vi "mecanum-drive-pose-est-test.vi"(8 "error in (no error)":errorcluster) -> (0 "error out":errorcluster, 3 "Test Passed":bool)   [LabVIEW 2019]
uses:
  <vilib>/Rock Robotics/WPI/ThirdParty/JAS_Junk/TrajLib/MatBuilder_Create.vi
  <vilib>/Rock Robotics/WPI/ThirdParty/JAS_Junk/TrajLib/MatrixHelper_CoerceSize.vi
  <vilib>/Rock Robotics/WPI/ThirdParty/JAS_Junk/TrajLib/Util_CalcDist.vi
  <vilib>/Analysis/1siggen.llb/Gaussian White Noise.vi
  <vilib>/Rock Robotics/WPI/ThirdParty/JAS_Junk/TrajLib/Trajectory_Library.lvlib
panel:
  out "Upd Err":bool
  out "BenchProcessing Timer Per Pass":dbl
  out "BenchTotalTime":dbl
  out "BenchTotalPasses":dbl
  out "MaxErrPassed":bool
  out "TotalPassed":bool
  out "EerrSumNormalized":dbl
  out "Error Sum":dbl
  out "Max Error":dbl
  out "Using Vision":bool
  in  "UseVIsion":bool=TRUE
  out "VIsionUpdates":i32
  out "TotalTImeSecs":dbl
  out "Position Graph":cluster{dbl[], dbl[]}[](graph)
  out "PoesEstCreateErr":errorcluster
  # "< 0.125"
  # "< 0.05"
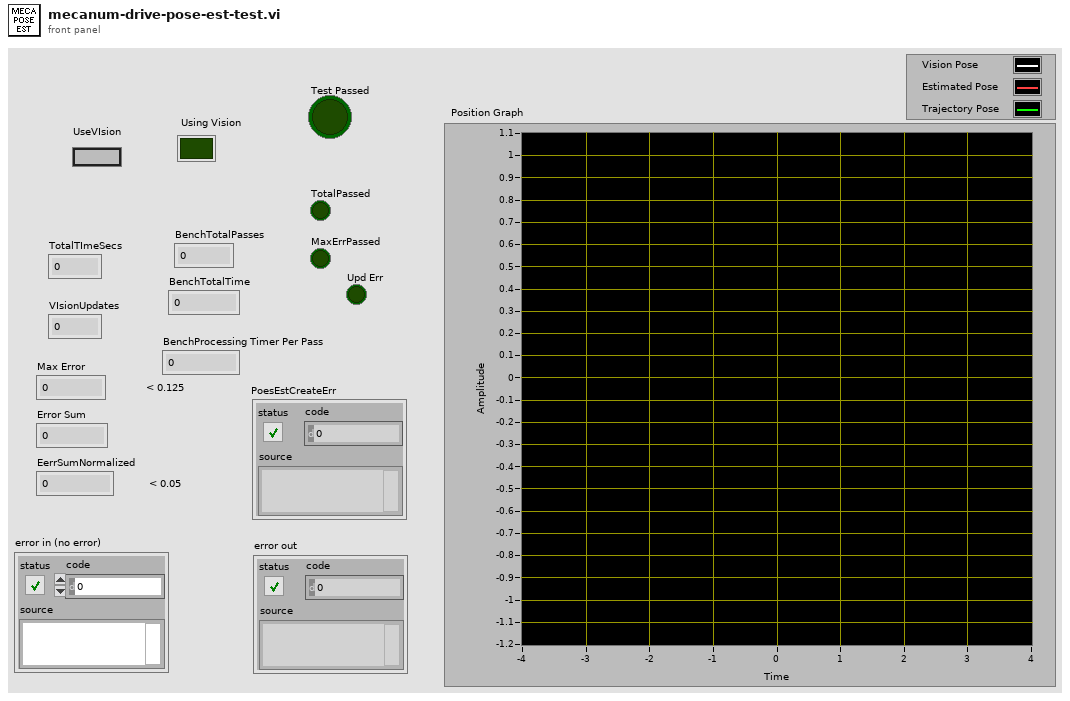
[diagram p1: front panel]
types:
  T1 = typedef "Trajectory_Library.lvlib/TRANSLATION2D.ctl" = cluster{"X":dbl, "Y":dbl}
  T2 = typedef "Trajectory_Library.lvlib/MECA_WHEEL_POSITIONS.ctl" = cluster{"FrontLeft":dbl, "FrontRight":dbl, "RearLeft":dbl, "RearRight":dbl, "P":bool}
  T3 = typedef "Trajectory_Library.lvlib/ROTATION2D.ctl" = cluster{"VALUE":dbl, "COS":dbl, "SIN":dbl}
  T4 = typedef "Trajectory_Library.lvlib/POSE2D.ctl" = cluster{"TRANSLATION":T1, "ROTATION":T3}
  T5 = typedef "NI_Matrix.lvlib/RealMatrix.ctl" = dbl[][]
  T6 = typedef "Trajectory_Library.lvlib/MECA_DRIVE_KINEMATICS.ctl" = cluster{"FrontLeft":T1, "FrontRight":T1, "RearLeft":T1, "RearRight":T1, "InverseKinematics":T5, "ForwardKinematics":T5, "PrevCoR":T1}
  T7 = typedef "Trajectory_Library.lvlib/TRAJ_CONFIG.ctl" = cluster{"MaxVelocity":dbl, "Max Acceleration":dbl, "StartVelocity":dbl, "End Velocity":dbl, "Reversed":bool, "Constraints":variant[]}
  T8 = typedef "Trajectory_Library.lvlib/MECA_DRIVE_POSE_EST.ctl" = cluster{"M_VisionContR":T5, "m_nominal_dT":dbl, "m_PrevTime_Sec":dbl, "m_GyroOffset":T3, "m_PrevAngle":T3, "m_Observer":T9, "m_kinematics":T6, "Pose_Buffer":T12}
  T9 = typedef "Trajectory_Library.lvlib/UNSCENTED_KALMAN_FILTER.ctl" = cluster{"m_P":T5, "m_xHat":T5, "States":i32, "Outputs":i32, "m_ContR":T5, "m_ContQ":T5, "m_SigmasF":T5, "m_dT_Sec":dbl, "MERWE_SCALED_SIGMA_PTS":T10, "meanFuncX":T11, "meanFuncY":T11, "residualFuncX":T11, "residualFuncY":T11, "addFuncX":T11, "addFuncXExtra":variant, "residualFuncYExtra":variant, "residualFuncXExtra":variant, "MeanFuncYExtra":variant, "MeanFuncXExtra":variant, "Inputs":i32}
  T10 = typedef "Trajectory_Library.lvlib/MERWE_SCALED_SIGMA_PTS.ctl" = cluster{"m_Wm":T5, "States":i32, "Alpha":dbl, "m_Wc":T5, "Kappa":i32}
  T11 = typedef "Trajectory_Library.lvlib/CALLBACK_FUNC_TYPE.ctl" = refnum<vi>
  T12 = typedef "Trajectory_Library.lvlib/TIME_INTERPOLATABLE_POSE2D.ctl" = cluster{"TimeStamps":dbl[], "Pose":T4[], "Min_TimeStamp":dbl, "Max_TimeStamp":dbl, "ItemCount":i32, "MaxBufferTime":dbl}
  T13 = typedef "Trajectory_Library.lvlib/TRAJECTORY.ctl" = cluster{"TotalTImeSecs":dbl, "States":T14[]}
  T14 = typedef "Trajectory_Library.lvlib/TRAJ_STATE.ctl" = cluster{"TimeSeconds":dbl, "Velocity":dbl, "Acceleration":dbl, "POSE":T4, "Curvature":dbl}
  T15 = typedef "Trajectory_Library.lvlib/CHASSIS_SPEEDS.ctl" = cluster{"vX":dbl, "vY":dbl, "vOmega":dbl}
  T16 = typedef "Trajectory_Library.lvlib/MECA_WHEEL_SPEEDS.ctl" = cluster{"FrontLeftSpeed":dbl, "FrontRightSpeed":dbl, "RearLeftSpeed":dbl, "RearRightSpeed":dbl}
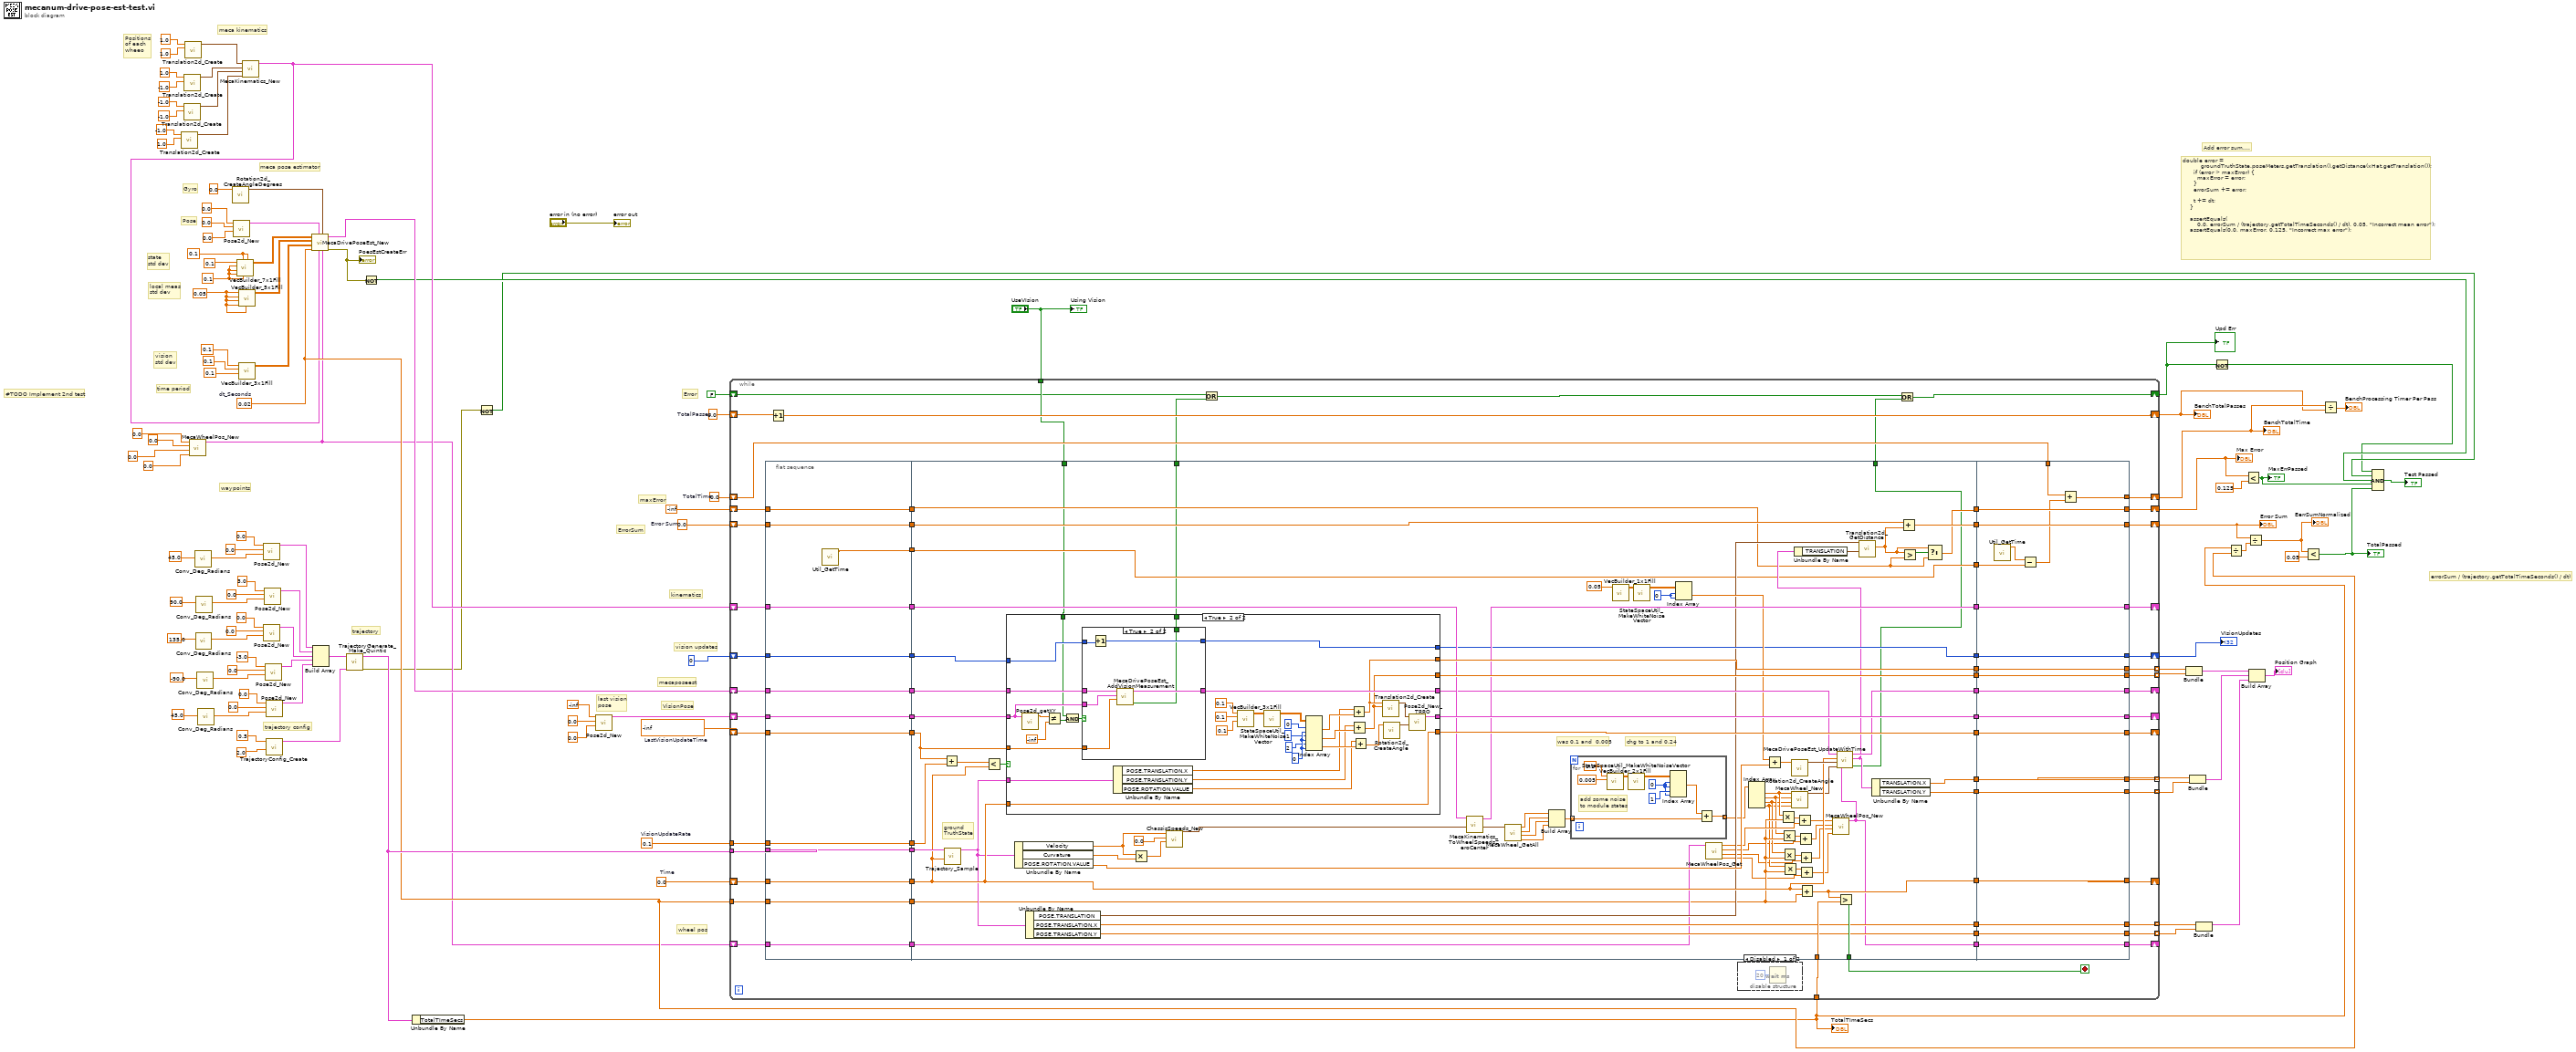
[diagram p0: block diagram]
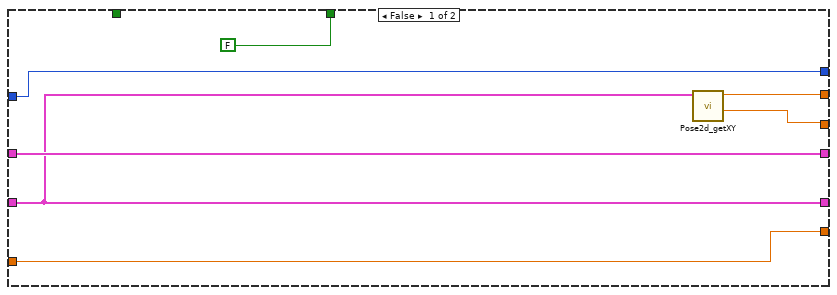
[diagram p3: hidden frame]
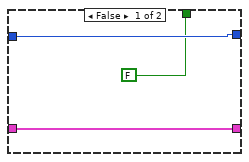
[diagram p4: hidden frame]
diagram:
  w24 = 0.0  # TotalPasses
  w25 = 0.0  # TotalTime
  w37 = 0.0  # Error Sum
  w55 = 0.1  # VisionUpdateRate
  w56 = -inf  # LastVisionUpdateTime
  w58 = 0.0  # Time
  w35 = 0.02  # dt_Seconds
  w8 = 0.05 ("element")
  w9 = 0.1 ("element")
  w11 = 0.1 ("element")
  # "#TODO Implement 2nd test"
  # "errorSum / (trajectory.getTotalTimeSeconds() / dt)"
  # "Error"
  # "Add error sum...."
  # "double error =\n          groundTruthState.poseMeters.getTranslation().getDistance(xHat.getTranslation());\n      if (error > maxError) {\n        maxError = error;\n      }\n      errorSum += error;\n\n      t += dt;\n    }\n\n    assertEquals(\n        0.0, errorSum / (trajectory.getTotalTimeSeconds() / dt), 0.05, \"Incorrect mean error\");\n    assertEquals(0.0, maxError, 0.125, \"Incorrect max error\");"
  # "wheel pos"
  # "ErrorSum"
  # "maxError"
  # "vision updates"
  # "kinematics"
  # "mecaposeest"
  # "VisionPose"
  # "last vision\npose"
  # "time period"
  # "vision \nstd dev"
  # "local meas\nstd dev"
  # "state\nstd dev"
  # "Pose"
  # "Gyro"
  # "Positions\nof each\nwheeo"
  # "meca pose estimator"
  # "meca kinematics"
  # "trajectory config"
  # "trajectory"
  # "waypoints"
  n1 = call <vilib>:"Translation2d_Create.vi"("Y"=1.0, "X"=-1.0) -> ("TRANSLATION"=w71:T1)  [unwired: 9 in]
  n2 = call <vilib>:"Translation2d_Create.vi"("Y"=-1.0, "X"=-1.0) -> ("TRANSLATION"=w72:T1)  [unwired: 9 in]
  n3 = call <vilib>:"Translation2d_Create.vi"("Y"=-1.0, "X"=1.0) -> ("TRANSLATION"=w73:T1)  [unwired: 9 in]
  n4 = call <vilib>:"Translation2d_Create.vi"("Y"=1.0, "X"=1.0) -> ("TRANSLATION"=w74:T1)  [unwired: 9 in]
  n5 = call <vilib>:"MecaWheelPos_New.vi"("RearRightPosition"=0.0, "RearLeftPosition"=0.0, "FrontRightPosition"=0.0, "FrontLeftPosition"=0.0) -> ("MECA_WHEEL_POSITIONS"=w12:T2)  [unwired: 7 in]
  n6 = call <vilib>:"Conv_Deg_Radians.vi"("Degress"=45.0 ("Heading")) -> ("Radians"=w88:dbl)  [unwired: 10 in]
  n7 = call <vilib>:"Conv_Deg_Radians.vi"("Degress"=135.0 ("Heading")) -> ("Radians"=w96:dbl)  [unwired: 10 in]
  n8 = call <vilib>:"Conv_Deg_Radians.vi"("Degress"=90.0 ("Heading")) -> ("Radians"=w92:dbl)  [unwired: 10 in]
  n9 = call <vilib>:"Conv_Deg_Radians.vi"("Degress"=-90.0 ("Heading")) -> ("Radians"=w100:dbl)  [unwired: 10 in]
  n10 = call <vilib>:"Conv_Deg_Radians.vi"("Degress"=45.0 ("Heading")) -> ("Radians"=w104:dbl)  [unwired: 10 in]
  n11 = call <vilib>:"Rotation2d_CreateAngleDegrees.vi"("Angle_Degrees"=0.0) -> ("ROTATION"=w70:T3)  [unwired: 10 in]
  n12 = call <vilib>:"Pose2d_New.vi"("Heading"=0.0, "Y"=0.0, "X"=0.0) -> ("out POSe"=w68:T4)  [unwired: 8 in]
  n13 = call <vilib>:"VecBuilder_7x1Fill.vi"("R0"=w11, "R6"=w9, "R1"=w11, "R5"=w9, "R4"=w9, "R3"=w9, "R2"=0.1 ("element")) -> ("output matrix"=w64:T5)  [unwired: 4 in]
  n14 = call <vilib>:"VecBuilder_5x1Fill.vi"("R4"=w8, "R3"=w8, "R2"=w8, "R1"=w8, "R0"=w8) -> ("output matrix"=w63:T5)  [unwired: 6 in]
  n15 = call <vilib>:"VecBuilder_3x1Fill.vi"("R2"=0.1 ("element"), "R1"=0.1 ("element"), "R0"=0.1 ("element")) -> ("output matrix"=w59:T5)  [unwired: 8 in]
  n16 = call <vilib>:"MecaKinematics_New.vi"("RearRight"=w71, "RearLeft"=w72, "FrontRight"=w73, "FrontLeft"=w74) -> ("MECA_DRIVE_KINEMATICS"=w17:T6)  [unwired: 7 in]
  n17 = call <vilib>:"Pose2d_New.vi"("Heading"=w88, "Y"=0.0, "X"=0.0) -> ("out POSe"=w87:T4)  [unwired: 8 in]
  n18 = call <vilib>:"Pose2d_New.vi"("Heading"=w96, "Y"=0.0, "X"=0.0) -> ("out POSe"=w84:T4)  [unwired: 8 in]
  n19 = call <vilib>:"Pose2d_New.vi"("Heading"=w92, "Y"=0.0, "X"=3.0) -> ("out POSe"=w85:T4)  [unwired: 8 in]
  n20 = call <vilib>:"Pose2d_New.vi"("Heading"=w100, "Y"=0.0, "X"=-3.0) -> ("out POSe"=w83:T4)  [unwired: 8 in]
  n21 = call <vilib>:"Pose2d_New.vi"("Heading"=w104, "Y"=0.0, "X"=0.0) -> ("out POSe"=w109:T4)  [unwired: 8 in]
  n22 = call <vilib>:"TrajectoryConfig_Create.vi"("MaxAcceleration"=2.0, "MaxVelocity"=0.5) -> ("TRAJECTORY_CONFIG"=w106:T7)  [unwired: 9 in]
  n23 = call <vilib>:"MecaDrivePoseEst_New.vi"("WheelPositions"=w12, "gyroAngle"=w70, "MecanumKinematics"=w17, "InitialPose"=w68, "dt_Seconds"=w35, "VisionMeasurementStdDevs"=w59, "LocalMeasurementStdDevs"=w63, "StateStdDevs"=w64) -> ("Error"=w7:errorcluster, "MecaDrivePoseEstimate"=w18:T8)  [unwired: 2 in]
  "PoesEstCreateErr" <- w7
  n24 = Build Array(w87, w85, w84, w83, w109) -> (w107:T4[])
  n25 = call <vilib>:"TrajectoryGenerate_Make_Quintic.vi"("traj_config"=w106, "waypointPOSE"=w107) -> ("error out"=w5:errorcluster, "TRAJECTORY"=w57:T13)  [unwired: 8 in]
  n26 = Not(x=w7) -> (.not. x?=w6:bool)
  n27 = Unbundle By Name(w57) -> ("TotalTImeSecs"=w28:dbl)
  "TotalTImeSecs" <- w28
  n28 = Not(x=w5) -> (.not. x?=w4:bool)
  n29 = call <vilib>:"Pose2d_New.vi"("Heading"=0.0, "Y"=0.0, "X"=-inf) -> ("out POSe"=w51:T4)  [unwired: 8 in]
  n30 = while {
    tunnel: w35 -> [w179]
    shift-right: [w178] -> _
    shift-left: w58 -> [w165]
    tunnel: w57 -> [w176]
    tunnel: w28 -> [w177]
    shift-right: [w170] -> _
    shift-left: w56 -> [w172]
    tunnel: w55 -> [w175]
    shift-right: [w171] -> _
    shift-left: w51 -> [w174]
    shift-right: [w164] -> _
    shift-left: w18 -> [w173]
    tunnel: [w169] -> w50 mode=indexing
    tunnel: [w168] -> w49 mode=indexing
    shift-right: [w166] -> _
    shift-left: w17 -> [w167]
    tunnel: [w163] -> w48 mode=indexing
    tunnel: [w162] -> w47 mode=indexing
    shift-right: [w160] -> w42
    shift-left: 0 -> [w161]
    tunnel: [w159] -> w41 mode=indexing
    tunnel: [w158] -> w40 mode=indexing
    shift-right: [w155] -> w33
    shift-left: -inf -> [w154]
    shift-right: [w156] -> w36
    shift-left: w37 -> [w157]
    shift-right: [w125] -> w23
    shift-left: w25 -> [w124]
    shift-right: [w122] -> w22
    shift-left: w24 -> [w123]
    tunnel: "UseVIsion" -> [w121]
    shift-right: [w117] -> _
    shift-left: w12 -> [w120]
    shift-right: [w112] -> w2
    shift-left: FALSE -> [w115]
    stop <- w153 stop-if-true
    n31 = flat-sequence {
      tunnel: w154 -> [w183]
      tunnel: w157 -> [w184]
      tunnel: w161 -> [w185]
      tunnel: w165 -> [w186]
      tunnel: w167 -> [w187]
      tunnel: w172 -> [w188]
      tunnel: w173 -> [w189]
      tunnel: w174 -> [w190]
      tunnel: w175 -> [w191]
      tunnel: w176 -> [w192]
      tunnel: w179 -> [w193]
      tunnel: [w193] -> w152
      tunnel: [w192] -> w151
      tunnel: [w191] -> w150
      tunnel: [w190] -> w149
      tunnel: [w189] -> w148
      tunnel: [w188] -> w147
      tunnel: [w187] -> w146
      tunnel: [w186] -> w145
      tunnel: [w185] -> w144
      tunnel: [w184] -> w143
      tunnel: [w183] -> w142
      tunnel: [w182] -> w127
      tunnel: w120 -> [w181]
      tunnel: [w181] -> w119
      tunnel: [w272] -> w153
      tunnel: w177 -> [w270]
      tunnel: w152 -> [w207]
      tunnel: w151 -> [w269]
      tunnel: w150 -> [w267]
      tunnel: w149 -> [w265]
      tunnel: w148 -> [w264]
      tunnel: w147 -> [w263]
      tunnel: w146 -> [w253]
      tunnel: w145 -> [w242]
      tunnel: w144 -> [w238]
      tunnel: w143 -> [w230]
      tunnel: w142 -> [w225]
      tunnel: [w271] -> w141
      tunnel: [w262] -> w140
      tunnel: [w261] -> w139
      tunnel: [w260] -> w138
      tunnel: [w259] -> w137
      tunnel: [w252] -> w136
      tunnel: [w241] -> w135
      tunnel: [w240] -> w134
      tunnel: [w239] -> w133
      tunnel: [w237] -> w132
      tunnel: [w235] -> w131
      tunnel: [w234] -> w130
      tunnel: [w229] -> w129
      tunnel: [w226] -> w128
      tunnel: w127 -> [w224]
      tunnel: [w224] -> w126
      tunnel: w121 -> [w223]
      tunnel: w119 -> [w214]
      tunnel: [w196] -> w118
      tunnel: [w195] -> w116
      tunnel: [w194] -> w114
      tunnel: [w340] -> w155
      tunnel: [w341] -> w156
      tunnel: [w342] -> w158
      tunnel: [w343] -> w159
      tunnel: [w344] -> w160
      tunnel: [w345] -> w162
      tunnel: [w346] -> w163
      tunnel: [w347] -> w164
      tunnel: [w348] -> w166
      tunnel: [w349] -> w168
      tunnel: [w350] -> w169
      tunnel: [w351] -> w170
      tunnel: [w352] -> w171
      tunnel: [w353] -> w178
      tunnel: w141 -> [w353]
      tunnel: w140 -> [w352]
      tunnel: w139 -> [w351]
      tunnel: w138 -> [w350]
      tunnel: w137 -> [w349]
      tunnel: w136 -> [w348]
      tunnel: w135 -> [w347]
      tunnel: w134 -> [w346]
      tunnel: w133 -> [w345]
      tunnel: w132 -> [w344]
      tunnel: w131 -> [w343]
      tunnel: w130 -> [w342]
      tunnel: w129 -> [w341]
      tunnel: w128 -> [w340]
      tunnel: w126 -> [w338]
      tunnel: [w337] -> w125
      tunnel: w124 -> [w335]
      tunnel: w118 -> [w334]
      tunnel: [w334] -> w117
      frame #0 {
        n32 = call <vilib>:"Util_GetTime.vi"() -> ("FPGA_Time_Seconds"=w182:dbl)  [unwired: 10 in, 1 out]
      }
      frame #1 {
        w247 = 0 ("index (col)")
        # "chg to 1 and 0.24"
        # "was 0.1 and  0.005"
        # "ground\nTruthState"
        n33 = Add(x=w263, y=w267) -> (x+y=w266:dbl)
        n34 = call <vilib>:"Trajectory_Sample.vi"("Time"=w242, "InputTRAJECTORY"=w269) -> ("OutputTRAJ_STATE"=w236:T14)  [unwired: 9 in]
        n35 = Less?(x=w266, y=w242) -> (x < y?=w268:bool)
        n36 = case shown="True" w268 {
          tunnel: w265 -> [w286 w320]
          tunnel: w264 -> [w288 w321]
          tunnel: [w288 w319] -> w251
          tunnel: w263 -> [w287 w318]
          tunnel: w236 -> [_ w311]
          tunnel: [w286 w317] -> w262
          tunnel: w242 -> [_ w297]
          tunnel: [w287 w297] -> w261
          tunnel: [w285 w296] -> w260
          tunnel: [w284 w295] -> w259
          tunnel: w238 -> [w283 w294]
          tunnel: [w283 w293] -> w237
          tunnel: w223 -> [_ w290]
          tunnel: [FALSE w289] -> w195
          frame False {
            n37 = call <vilib>:"Pose2d_getXY.vi"("in POSE"=w286) -> ("Y"=w284:dbl, "X"=w285:dbl)  [unwired: 9 in]
          }
          frame True {
            w308 = 0 ("index (col)")
            n38 = call <vilib>:"Pose2d_getXY.vi"("in POSE"=w320) -> ("X"=w323:dbl)  [unwired: 9 in, 1 out]
            n39 = Not Equal?(x=w323, y=-inf) -> (x != y?=w291:bool)
            n40 = And(x=w290, y=w291) -> (x .and. y?=w292:bool)
            n41 = case shown="True" w292 {
              tunnel: w321 -> [w326 w333]
              tunnel: w320 -> [_ w332]
              tunnel: [w326 w331] -> w319
              tunnel: w318 -> [_ w330]
              tunnel: w294 -> [w325 w329]
              tunnel: [w325 w328] -> w293
              tunnel: [FALSE w327] -> w289
              frame False {
              }
              frame True {
                n42 = Increment(x=w329) -> (x+1=w328:i32)
                n43 = call <vilib>:"MecaDrivePoseEst_AddVisionMeasurement.vi"("TImeStamp_Seconds"=w330, "visionRobotPose"=w332, "in MecaDrivePoseEstimate"=w333) -> ("Error"=w327:bool, "OutMecaDrivePoseEstimate"=w331:T8)  [unwired: 7 in]
              }
            }
            n44 = Unbundle By Name(w311) -> ("POSE.TRANSLATION.X"=w300:dbl, "POSE.TRANSLATION.Y"=w299:dbl, "POSE.ROTATION.VALUE"=w298:dbl)
            n45 = call <vilib>:"VecBuilder_3x1Fill.vi"("R2"=0.1, "R1"=0.1, "R0"=0.1) -> ("output matrix"=w315:T5)  [unwired: 8 in]
            n46 = call <vilib>:"StateSpaceUtil_MakeWhiteNoiseVector.vi"("StdDevs"=w315) -> ("WhiteNoise"=w309:T5)  [unwired: 9 in, 1 out]
            n47 = Index Array(array=w309, index (row) #1=0 ("index (col)"), index (col) #1=w308, index (row) #2=1 ("index (col)"), index (col) #2=w308, index (row) #3=2 ("index (col)"), index (col) #3=w308) -> (element #1=w302:dbl, element #2=w303:dbl, element #3=w304:dbl)
            n48 = Add(x=w300, y=w302) -> (x+y=w296:dbl)
            n49 = Add(x=w299, y=w303) -> (x+y=w295:dbl)
            n50 = Add(x=w298, y=w304) -> (x+y=w301:dbl)
            n51 = call <vilib>:"Translation2d_Create.vi"("Y"=w295, "X"=w296) -> ("TRANSLATION"=w316:T1)  [unwired: 9 in]
            n52 = call <vilib>:"Rotation2d_CreateAngle.vi"("Angle"=w301) -> ("ROTATION"=w310:T3)  [unwired: 10 in]
            n53 = call <vilib>:"Pose2d_New_TRRO.vi"("ROTATION"=w310, "TRANSLATION"=w316) -> ("outPOSE"=w317:T4)  [unwired: 9 in]
          }
        }
        n54 = Unbundle By Name(w236) -> ("Velocity"=w256:dbl, "Curvature"=w257:dbl, "POSE.ROTATION.VALUE"=w246:dbl)
        n55 = Unbundle By Name(w236) -> ("POSE.TRANSLATION"=w233:T1, "POSE.TRANSLATION.X"=w234:dbl, "POSE.TRANSLATION.Y"=w235:dbl)
        n56 = Multiply(x=w256, y=w257) -> (x*y=w255:dbl)
        n57 = call <vilib>:"ChassisSpeeds_New.vi"("vAngular"=w255, "vY"=0.0, "vX"=w256) -> ("CHASSIS"=w254:T15)  [unwired: 8 in]
        n58 = call <vilib>:"MecaKinematics_ToWheelSpeedsZeroCenter.vi"("ChassisSpeeds"=w254, "in MECA_DRIVE_KINEMATICS"=w253) -> ("MECA_WHEEL_SPEEDS"=w222:T16, "out MECA_DRIVE_KINEMATICS"=w252:T6)  [unwired: 8 in]
        n59 = call <vilib>:"MecaWheel_GetAll.vi"("MECA_WHEEL_SPEEDS"=w222) -> ("RearRightSpeed"=w218:dbl, "RearLeftSpeed"=w219:dbl, "FrontRightSpeed"=w220:dbl, "FrontLeftSpeed"=w221:dbl)  [unwired: 7 in]
        n60 = Build Array(w221, w220, w219, w218) -> (w217:dbl[])
        n61 = for {
          tunnel: [w273] -> w216 mode=indexing
          tunnel: w217 -> [w274] mode=indexing
          w276 = 0 ("index (col)")
          # "add some noise\nto module states"
          n62 = call <vilib>:"VecBuilder_2x1Fill.vi"("R1"=0.005, "R0"=0.1) -> ("output matrix"=w281:T5)  [unwired: 9 in]
          n63 = call <vilib>:"StateSpaceUtil_MakeWhiteNoiseVector.vi"("StdDevs"=w281) -> ("WhiteNoise"=w278:T5)  [unwired: 9 in, 1 out]
          n64 = Index Array(array=w278, index (row) #1=w276, index (col) #1=w276, index (row) #2=1 ("index (col)"), index (col) #2=w276) -> (element #1=w275:dbl)  [unwired: 1 out]
          n65 = Add(x=w275, y=w274) -> (x+y=w273:dbl)
        }
        n66 = call <vilib>:"VecBuilder_1x1Fill.vi"("R0_C0"=0.05 ("R0")) -> ("output matrix"=w250:T5)  [unwired: 10 in]
        n67 = call <vilib>:"StateSpaceUtil_MakeWhiteNoiseVector.vi"("StdDevs"=w250) -> ("WhiteNoise"=w248:T5)  [unwired: 9 in, 1 out]
        n68 = Index Array(array=w248, index (row)=w247, index (col)=w247) -> (element=w245:dbl)
        n69 = call <vilib>:"MecaWheelPos_Get.vi"("MECA_WHEEL_POSITIONS"=w214) -> ("RearRightPosition"=w201:dbl, "RearLeftPosition"=w202:dbl, "FrontRightPosition"=w203:dbl, "FrontLeftPosition"=w212:dbl)  [unwired: 7 in]
        n70 = Index Array(array=w216) -> (element #1=w208:dbl, element #2=w206:dbl, element #3=w205:dbl, element #4=w204:dbl)  [unwired: 4 in]
        n71 = Add(x=w245, y=w246) -> (x+y=w244:dbl)
        n72 = Multiply(x=w208, y=w207) -> (x*y=w213:dbl)
        n73 = Multiply(x=w206, y=w207) -> (x*y=w211:dbl)
        n74 = Multiply(x=w205, y=w207) -> (x*y=w210:dbl)
        n75 = Multiply(x=w204, y=w207) -> (x*y=w209:dbl)
        n76 = call <vilib>:"Rotation2d_CreateAngle.vi"("Angle"=w244) -> ("ROTATION"=w243:T3)  [unwired: 10 in]
        n77 = call <vilib>:"MecaWheel_New.vi"("RearRightSpeed"=w204, "RearLeftSpeed"=w205, "FrontRightSpeed"=w206, "FrontLeftSpeed"=w208) -> ("MECA_WHEEL_SPEEDS"=w215:T16)  [unwired: 7 in]
        n78 = Add(x=w213, y=w212) -> (x+y=w200:dbl)
        n79 = Add(x=w211, y=w203) -> (x+y=w199:dbl)
        n80 = Add(x=w210, y=w202) -> (x+y=w198:dbl)
        n81 = Add(x=w209, y=w201) -> (x+y=w197:dbl)
        n82 = Add(x=w242, y=w207) -> (x+y=w271:dbl)
        n83 = call <vilib>:"MecaWheelPos_New.vi"("RearRightPosition"=w197, "RearLeftPosition"=w198, "FrontRightPosition"=w199, "FrontLeftPosition"=w200) -> ("MECA_WHEEL_POSITIONS"=w196:T2)  [unwired: 7 in]
        n84 = call <vilib>:"MecaDrivePoseEst_UpdateWithTime.vi"("MecanumWheelPositions"=w196, "MecanumWheelSpeeds"=w215, "GyroAngle"=w243, "CurrentTimeSeconds"=w242, "in MecaDrivePoseEstimate"=w251) -> ("Error"=w194:bool, "Estimated Pose"=w232:T4, "Out MecaDrivePoseEstimate"=w241:T8)  [unwired: 4 in]
        n85 = Unbundle By Name(w232) -> ("TRANSLATION"=w231:T1)
        n86 = Greater?(x=w271, y=w270) -> (0:w272:bool)
        n87 = call <vilib>:"Translation2d_GetDistance.vi"("other Translation"=w231, "In Translation"=w233) -> ("Distance"=w227:dbl)  [unwired: 9 in]
        n88 = Unbundle By Name(w232) -> ("TRANSLATION.X"=w240:dbl, "TRANSLATION.Y"=w239:dbl)
        n89 = Add(x=w230, y=w227) -> (x+y=w229:dbl)
        n90 = Greater?(x=w227, y=w225) -> (0:w228:bool)
        n91 = Select(t=w227, s=w228, f=w225) -> (s? t:f=w226:dbl)
      }
      frame #2 {
        n92 = call <vilib>:"Util_GetTime.vi"() -> ("FPGA_Time_Seconds"=w339:dbl)  [unwired: 10 in, 1 out]
        n93 = Subtract(x=w339, y=w338) -> (x-y=w336:dbl)
        n94 = Add(x=w335, y=w336) -> (x+y=w337:dbl)
      }
    }
    n95 = Increment(x=w123) -> (x+1=w122:dbl)
    n96 = Or(x=w115, y=w116) -> (x .or. y?=w113:bool)
    n97 = disable-structure shown="Disabled" {
      frame Disabled {
        n98 = Wait (ms)(milliseconds to wait=u32 20) -> ()  [unwired: 1 out]
      }
      frame Enabled {
      }
    }
    n99 = Or(x=w113, y=w114) -> (x .or. y?=w112:bool)
  }
  "VIsionUpdates" <- w42
  "Max Error" <- w33
  "Error Sum" <- w36
  "BenchTotalPasses" <- w22
  "BenchTotalTime" <- w23
  "Upd Err" <- w2
  n100 = Bundle(w50, w49) -> (w46:cluster{dbl[], dbl[]})  [unwired: 1 in]
  n101 = Bundle(w48, w47) -> (w45:cluster{dbl[], dbl[]})  [unwired: 1 in]
  n102 = Bundle(w40, w41) -> (w39:cluster{dbl[], dbl[]})  [unwired: 1 in]
  n103 = Not(x=w2) -> (.not. x?=w1:bool)
  n104 = Divide(x=w28, y=w35) -> (x/y=w26:dbl)
  n105 = Less?(x=w33, y=0.125) -> (x < y?=w31:bool)
  "MaxErrPassed" <- w31
  n106 = Divide(x=w36, y=w26) -> (x/y=w27:dbl)
  "EerrSumNormalized" <- w27
  n107 = Build Array(w46, w45, w39) -> (→"Position Graph":cluster{dbl[], dbl[]}[])
  n108 = Less?(x=w27, y=0.05) -> (x < y?=w30:bool)
  "TotalPassed" <- w30
  n109 = Divide(x=w23, y=w22) -> (x/y=→"BenchProcessing Timer Per Pass":dbl)
  n110 = Compound Arithmetic op=AND(w1, w4, w6, w31, w30) -> (→"Test Passed":bool)
  "Using Vision" <- "UseVIsion"
  "error out" <- "error in (no error)"
